vi "update spot.vi"(7 "dt":dbl=0.2, 10 "kalman result":T3, 11 "Spots":T2(array[cluster])=[{"pos"=[{"weighted sum"=0.0, "n measurements"=0.0, "t values"=[], "x values"=[], "t start"=0.0}, {"weighted sum"=0.0, "n measurements"=0.0, "t values"=[], "x values"=[], "t start"=0.0}, {"weighted sum"=0.0, "n measurements"=0.0, "t values"=[], "x values"=[], "t start"=0.0}], "red"={"weighted sum"=0.0, "n measurements"=0.0, "t values"=[], "x values"=[], "t start"=0.0}, "green"={"weighted sum"=0.0, "n measurements"=0.0, "t values"=[], "x values"=[], "t start"=0.0}, "ratio"={"weighted sum"=0.0, "n measurements"=0.0, "t values"=[], "x values"=[], "t start"=0.0}, "SPPF state"={"theta"=[], "w"=[], "elapsed time"=0.0}}]) -> (3 "spots out":T2(array[cluster]))   [LabVIEW 2010]
uses:
  kalman_result_scaled.ctl
panel:
  in  "default spot":T1={"pos"=[{"weighted sum"=0.0, "n measurements"=0.0, "t values"=[], "x values"=[], "t start"=0.0}, {"weighted sum"=0.0, "n measurements"=0.0, "t values"=[], "x values"=[], "t start"=0.0}, {"weighted sum"=0.0, "n measurements"=0.0, "t values"=[], "x values"=[], "t start"=0.0}], "red"={"weighted sum"=0.0, "n measurements"=0.0, "t values"=[], "x values"=[], "t start"=0.0}, "green"={"weighted sum"=0.0, "n measurements"=0.0, "t values"=[], "x values"=[], "t start"=0.0}, "ratio"={"weighted sum"=0.0, "n measurements"=0.0, "t values"=[], "x values"=[], "t start"=0.0}, "SPPF state"={"theta"=[0.0, 0.0], "w"=[[0.0, 0.0], [0.0, 0.0]], "elapsed time"=0.0}}
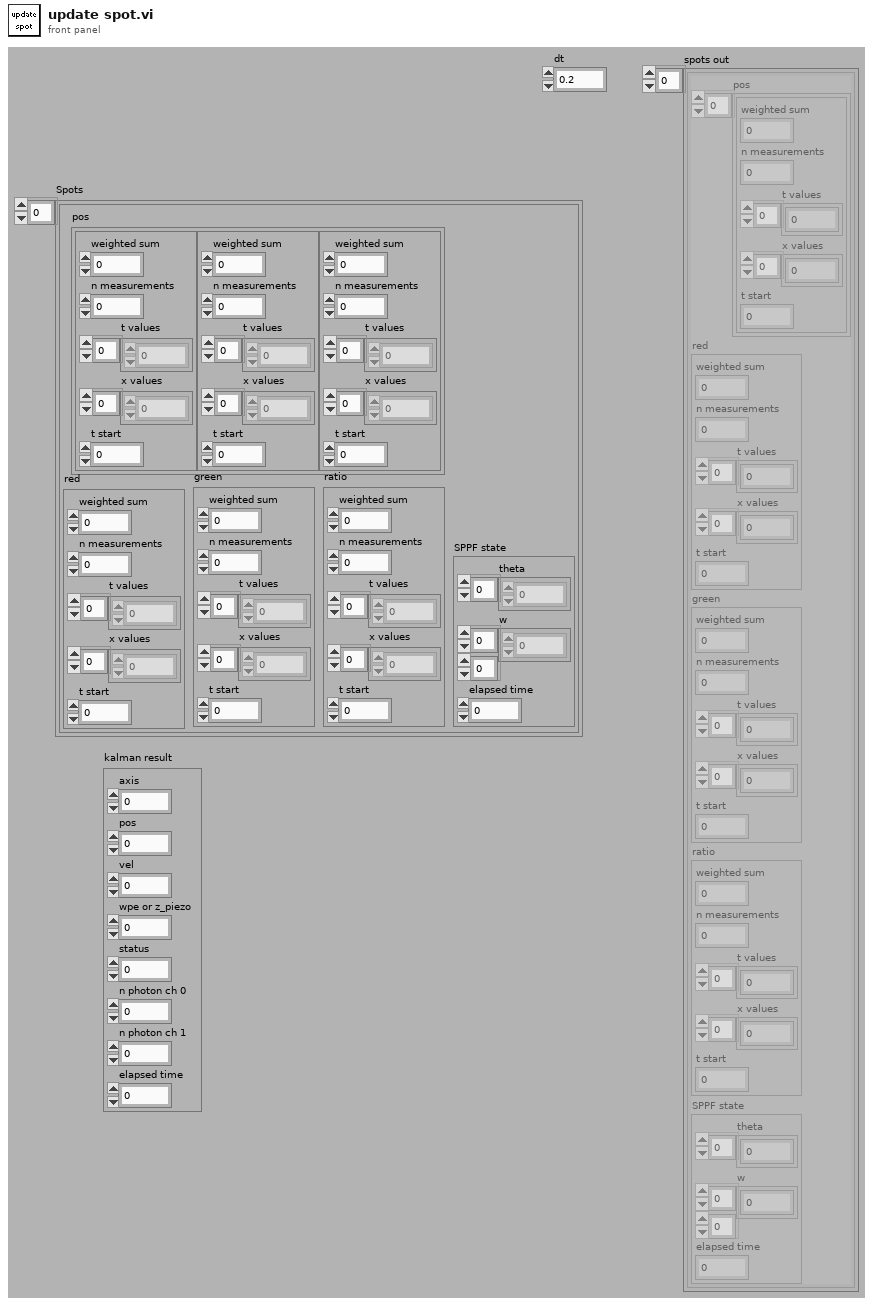
[diagram p1: front panel]
types:
  T1 = cluster{"pos":cluster{"weighted sum":dbl, "n measurements":dbl, "t values":dbl[], "x values":dbl[], "t start":dbl}[], "red":cluster{"weighted sum":dbl, "n measurements":dbl, "t values":dbl[], "x values":dbl[], "t start":dbl}, "green":cluster{"weighted sum":dbl, "n measurements":dbl, "t values":dbl[], "x values":dbl[], "t start":dbl}, "ratio":cluster{"weighted sum":dbl, "n measurements":dbl, "t values":dbl[], "x values":dbl[], "t start":dbl}, "SPPF state":cluster{"theta":dbl[], "w":dbl[][], "elapsed time":dbl}}
  T2 = cluster{"pos":cluster{"weighted sum":dbl, "n measurements":dbl, "t values":dbl[], "x values":dbl[], "t start":dbl}[], "red":cluster{"weighted sum":dbl, "n measurements":dbl, "t values":dbl[], "x values":dbl[], "t start":dbl}, "green":cluster{"weighted sum":dbl, "n measurements":dbl, "t values":dbl[], "x values":dbl[], "t start":dbl}, "ratio":cluster{"weighted sum":dbl, "n measurements":dbl, "t values":dbl[], "x values":dbl[], "t start":dbl}, "SPPF state":cluster{"theta":dbl[], "w":dbl[][], "elapsed time":dbl}}[]
  T3 = typedef "kalman_result_scaled.ctl" = cluster{"axis":u8, "pos":dbl, "vel":dbl, "wpe or z_piezo":dbl, "status":u32, "n photon ch 0":u32, "n photon ch 1":u32, "elapsed time":dbl}
  T4 = cluster{"theta":dbl[], "w":dbl[][], "elapsed time":dbl}
  T5 = cluster{"weighted sum":dbl, "n measurements":dbl, "t values":dbl[], "x values":dbl[], "t start":dbl}
  T6 = cluster{"weighted sum":dbl, "n measurements":dbl, "t values":dbl[], "x values":dbl[], "t start":dbl}[]
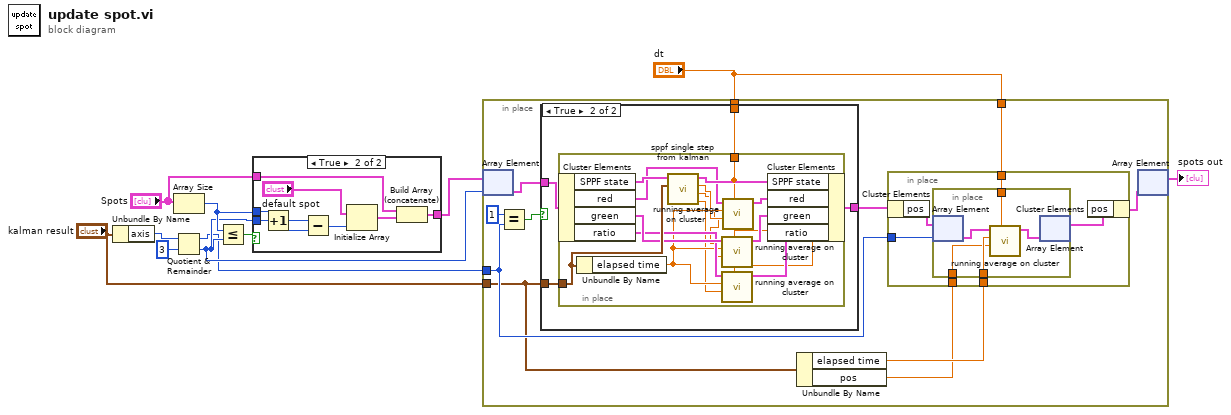
[diagram p0: block diagram]
diagram:
  n1 = Unbundle By Name("kalman result") -> ("axis"=w11:u8)
  n2 = Array Size(array="Spots") -> (size(s)=w8:i32)
  n3 = Quotient & Remainder(x=w11, y=u8 3) -> (x-y*floor(x/y)=w1:u8, floor(x/y)=w2:u8)
  n4 = Less Or Equal?(x=w8, y=w2) -> (x <= y?=w9:bool)
  n5 = case shown="True" w9 {
    tunnel: w2 -> [_ w20]
    tunnel: w8 -> [_ w19]
    tunnel: "Spots" -> [w12 w14]
    tunnel: [w12 w13] -> w6
    frame False {
    }
    frame True {
      n6 = Increment(x=w20) -> (x+1=w18:u8)
      n7 = Subtract(x=w18, y=w19) -> (x-y=w16:i32)
      n8 = Initialize Array("default spot", w16) -> (w15:T2)
      n9 = Build Array (concatenate)(w14, w15) -> (w13:T2)
    }
  }
  n10 = in-place {
    in-place-border: w1 -> [w28]
    in-place-border: "kalman result" -> [w27]
    in-place-border: "dt" -> [w23]
    in-place-border: "dt" -> [w22]
    n11 = in-place-array #1(w6, w2) -> (w31:T1)
    n12 = Equal?(x=u8 1, y=w28) -> (x = y?=w30:bool)
    n13 = case shown="True" w30 {
      tunnel: w31 -> [w43 w47]
      tunnel: w27 -> [_ w46]
      tunnel: [w43 w45] -> w29
      tunnel: w23 -> [_ w44]
      frame False {
      }
      frame True {
        n14 = in-place {
          in-place-border: w46 -> [w59]
          in-place-border: w44 -> [w51]
          n15 = in-place-cluster #2(w47) -> ("SPPF state"=w61:T4, "red"=w58:T5, "green"=w57:T5, "ratio"=w56:T5)
          n16 = Unbundle By Name(w59) -> ("elapsed time"=w55:dbl)
          n17 = call "sppf single step from kalman.vi"("kalman result"=w59, "SPPF state"=w61) -> ("ratio"=w50:dbl, "green rate"=w48:dbl, "red rate"=w49:dbl, "SPPF state out"=w60:T4)  [unwired: 3 in, 3 out]
          n18 = call "running average on cluster.vi"("dt"=w51, "x"=w48, "t"=w55, "averaging state cluster"=w57) -> ("averaging state cluster out"=w53:T5)  [unwired: 7 in]
          n19 = call "running average on cluster.vi"("dt"=w51, "x"=w50, "t"=w55, "averaging state cluster"=w56) -> ("averaging state cluster out"=w52:T5)  [unwired: 7 in]
          n20 = call "running average on cluster.vi"("dt"=w51, "x"=w49, "t"=w55, "averaging state cluster"=w58) -> ("averaging state cluster out"=w54:T5)  [unwired: 7 in]
          n21 = in-place-cluster #2("SPPF state"=w60, "red"=w54, "green"=w53, "ratio"=w52) -> (w45:T1)
        }
      }
    }
    n22 = Unbundle By Name(w27) -> ("elapsed time"=w26:dbl, "pos"=w25:dbl)
    n23 = in-place {
      in-place-border: w28 -> [w36]
      in-place-border: w26 -> [w35]
      in-place-border: w25 -> [w34]
      in-place-border: w22 -> [w32]
      n24 = in-place-cluster #3(w29) -> ("pos"=w37:T6)
      n25 = in-place {
        in-place-border: w35 -> [w41]
        in-place-border: w34 -> [w40]
        in-place-border: w32 -> [w38]
        n26 = in-place-array #4(w37, w36) -> (w42:T5)
        n27 = call "running average on cluster.vi"("dt"=w38, "x"=w40, "t"=w41, "averaging state cluster"=w42) -> ("averaging state cluster out"=w39:T5)  [unwired: 7 in]
        n28 = in-place-array #4(w39) -> (w33:T6)  [unwired: 1 out]
      }
      n29 = in-place-cluster #3("pos"=w33) -> (w24:T1)
    }
    n30 = in-place-array #1(w24) -> (→"spots out":T2)  [unwired: 1 out]
  }
